vi "Parse MKS Pressure String.vi"(8 "error in (no error)":errorcluster, 11 "String":string) -> (0 "error out":errorcluster, 3 "Pressure 1":dbl)   [LabVIEW 2020, in "MKS_PressureTransducer.lvclass"]
uses:
  MKS_PressureTransducer.lvclass
panel:
  out "substring":string
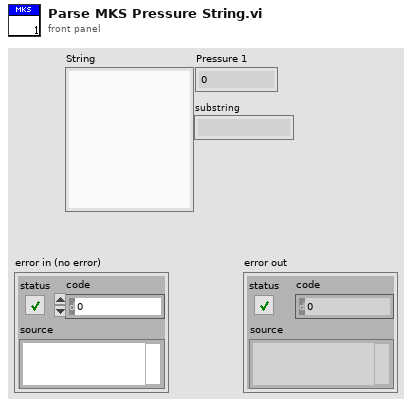
[diagram p1: front panel]
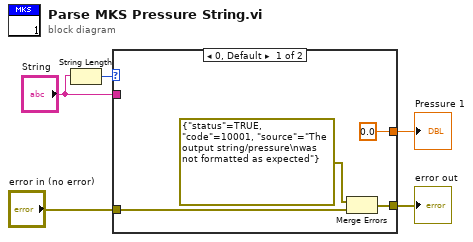
[diagram p0: block diagram]
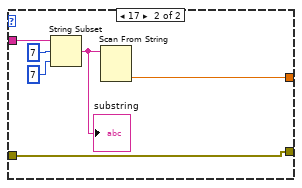
[diagram p2: hidden frame]
diagram:
  n1 = String Length(string="String") -> (length=w4:i32)
  n2 = case shown="0, Default" w4 {
    tunnel: "String" -> [_ w15]
    tunnel: "error in (no error)" -> [w9 w11]
    tunnel: [w8 w11] -> w2
    tunnel: [0.0 w10] -> w1
    frame 0, Default {
      n3 = Merge Errors(errorcluster {"status"=TRUE, "code"=10001, "source"="The output string/pressure\nwas not formatted as expected"} ("error in (no error)"), w9) -> (w8:errorcluster)
    }
    frame 17 {
      n4 = String Subset(string=w15, offset (0)=7, length (rest)=7 ("length (rest)")) -> (substring=w12:string)
      "substring" <- w12
      n5 = Scan From String(input string=w12) -> (output 1=w10:dbl)  [unwired: 4 in, 3 out]
    }
  }
  "error out" <- w2
  "Pressure 1" <- w1
